vi "Triggers Routing.vi"(7 "Function":enum16{"Connect routes", "Disconnect routes"}(ring), 8 "error in (no error)":errorcluster) -> (0 "error out (no error)":errorcluster)   [LabVIEW 2013]
uses:
  Typedefs/HW config states enum.ctl
  <vilib>/Utility/error.llb/DialogType.ctl
  Global Variables/General Globals.vi
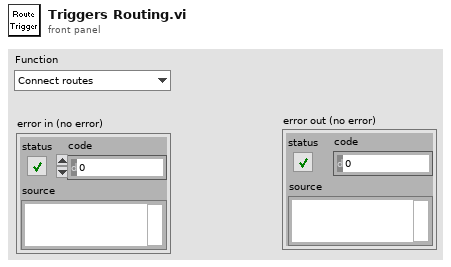
[diagram p1: front panel]
types:
  T1 = typedef "HW config states enum.ctl" = enum16{"Load from file", "Save to file", "Write all", "Read all", "Write XY stage settings", "Write DAQ FPGA settings", "Write Control FPGA settings", "Write Phys Channels", "Clear", "Compare from file"}
  T2 = typedef "Sys Configuration.ctl" = cluster{"XY Stage":T3, "DAQ FPGA":T4, "Control system":T8, "Encoder":T9, "DAQmx Chan":T10, "Computer MAC address":string, "Cam VidRec":T11, "Externalise Triggers":bool, "Laser wavelength (nm)":dbl}
  T3 = typedef "XY Stage config cluster.ctl" = cluster{"COM port":refnum<visa-resource-name>, "XY stage available":bool}
  T4 = typedef "DAQ FPGA config cluster.ctl" = cluster{"Ref":T5, "Target":T6, "Clock Freq (MHz) ":dbl, "input card type":T7, "Samples Wait after Trigger":u16, "AOD fill":u16, "StartupDelay":i32, "Slip Cycle (clock cycles)":u32, "Add Cycle":bool}
  T5 = typedef "FPGA Ref.ctl" = refnum<k20>
  T6 = typedef "nirio_resource_hc.ctl" = tag
  T7 = typedef "FPGA input type AC-DC.ctl" = enum16{"AC Card", "DC Card"}
  T8 = typedef "CTRL system config cluster.ctl" = cluster{"Ethernet opened":bool, "Ethernet Port":u32, "Ctrl FPGA available":bool, "Ctrl FPGA Clock (MHz)":dbl, "Ctrl system MAC address":string, "Control system.Network adapter name":string, "AOD 1 Amplitude":i16, "AOD 2 Amplitude":i16, "AOD 3 Amplitude":i16, "AOD 4 Amplitude":i16, "Data Time Interval (ns)":dbl, "T0 (ns)":dbl, "Ta (ns)":dbl}
  T9 = typedef "Encoder config cluster.ctl" = cluster{"IP address":string, "Port":u16, "Encoder available":bool, "Wheel radius (cm)":dbl}
  T10 = typedef "DAQmx physical channels cluster.ctl" = cluster{"Pockels AO":tag, "Hard shutter AO":tag, "PMT AOs":tag, "Power meter AI":tag}
  T11 = typedef "Cam VidRec HW config setup cluster.ctl" = cluster{"DO flag-Video record":tag, "DO flag-Trial start":tag, "VidRec available":bool}
  T12 = cluster{"PXI backplane trigger":tag, "PXI-6535 terminal to output trigger on":tag}[]
  T13 = typedef "Triggers output setup.ctl" = T14[]
  T14 = typedef "Trigger setup element cluster.ctl" = cluster{"Name":string, "Output?":bool, "Output terminal":tag, "PXI backplane line":tag, "Pulse width (us)":u16}
  T15 = typedef "DialogType.ctl" = u16
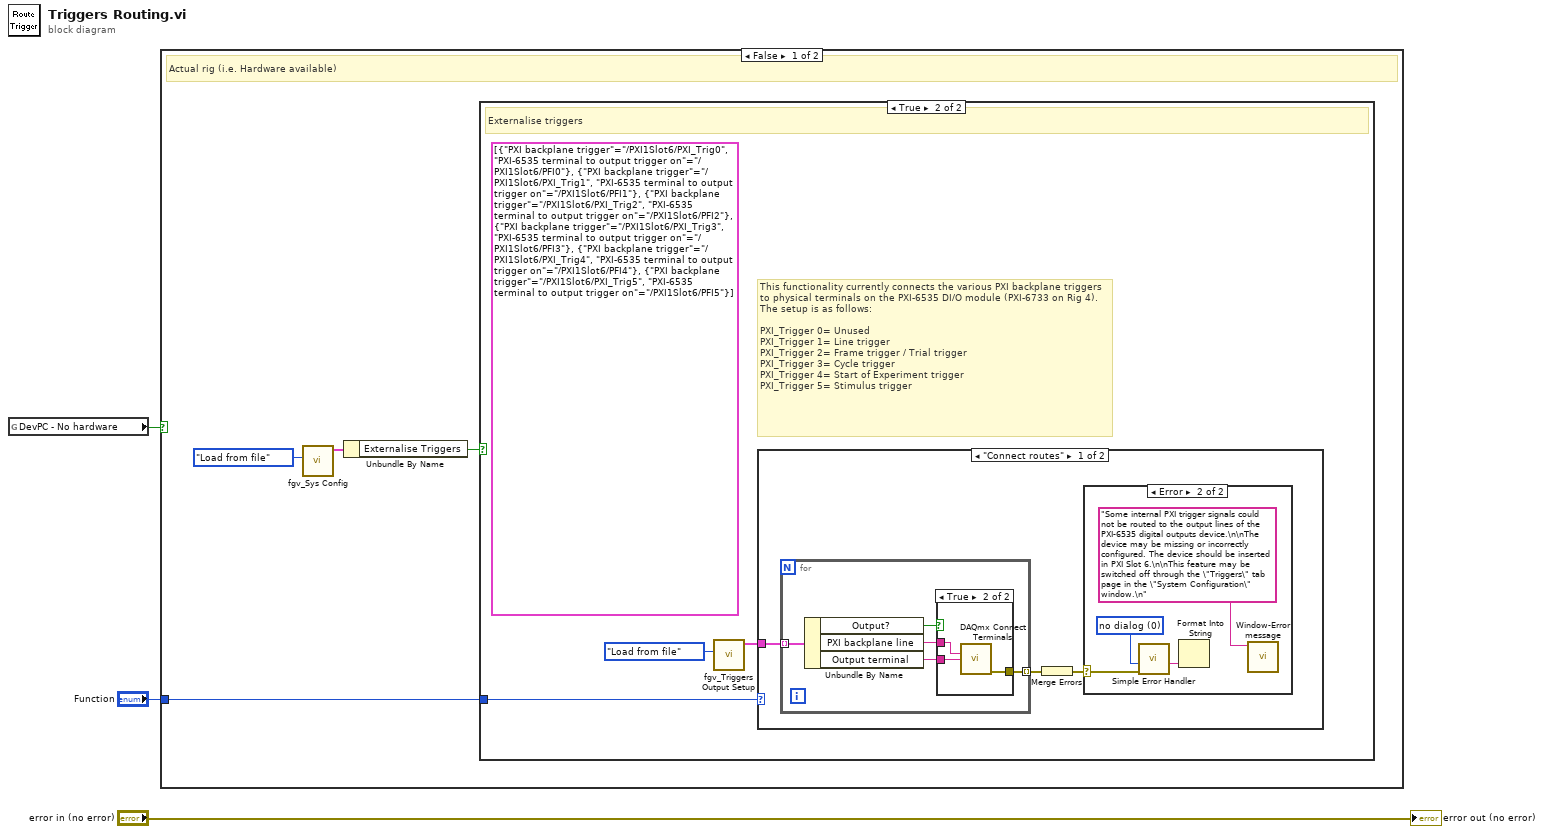
[diagram p0: block diagram]
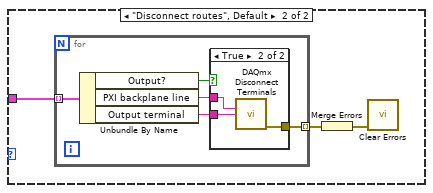
[diagram p5: hidden frame]
diagram:
  n1 = global read "General Globals.vi" "DevPC - No hardware"() -> (w1:bool)
  n2 = case shown="False" w1 {
    tunnel: "Function" -> [w4 _]
    frame False {
      # "Actual rig (i.e. Hardware available)"
      n3 = call "fgv_Sys Config.vi"("Function"=HW_config_states_enum."Load from file") -> ("System Config out"=w6:T2)  [unwired: 9 in, 1 out]
      n4 = Unbundle By Name(w6) -> ("Externalise Triggers"=w5:bool)
      n5 = case shown="True" w5 {
        tunnel: w4 -> [_ w8]
        frame False {
          # "\"Externalise triggers\" is OFF"
        }
        frame True {
          (unwired) T12 [{"PXI backplane trigger"="/PXI1Slot6/PXI_Trig0", "PXI-6535 terminal to output trigger on"="/PXI1Slot6/PFI0"}, {"PXI backplane trigger"="/PXI1Slot6/PXI_Trig1", "PXI-6535 terminal to output trigger on"="/PXI1Slot6/PFI1"}, {"PXI backplane trigger"="/PXI1Slot6/PXI_Trig2", "PXI-6535 terminal to output trigger on"="/PXI1Slot6/PFI2"}, {"PXI backplane trigger"="/PXI1Slot6/PXI_Trig3", "PXI-6535 terminal to output trigger on"="/PXI1Slot6/PFI3"}, {"PXI backplane trigger"="/PXI1Slot6/PXI_Trig4", "PXI-6535 terminal to output trigger on"="/PXI1Slot6/PFI4"}, {"PXI backplane trigger"="/PXI1Slot6/PXI_Trig5", "PXI-6535 terminal to output trigger on"="/PXI1Slot6/PFI5"}] ("Routes mapping array")
          # "This functionality currently connects the various PXI backplane triggers to physical terminals on the PXI-6535 DI/O module (PXI-6733 on Rig 4). The setup is as follows:\n\nPXI_Trigger 0= Unused\nPXI_Trigger 1= Line trigger\nPXI_Trigger 2= Frame trigger / Trial trigger\nPXI_Trigger 3= Cycle trigger\nPXI_Trigger 4= Start of Experiment trigger\nPXI_Trigger 5= Stimulus trigger"
          # "Externalise triggers"
          n6 = call "fgv_Triggers Output Setup.vi"("Function"=HW_config_states_enum."Load from file") -> ("Triggers output setup"=w10:T13)  [unwired: 9 in, 1 out]
          n7 = case shown="\"Connect routes\"" w8 {
            tunnel: w10 -> [w11 w26]
            frame "Connect routes" {
              n8 = for {
                tunnel: [w22] -> w13 mode=indexing
                tunnel: w11 -> [w19] mode=indexing
                n9 = Unbundle By Name(w19) -> ("Output?"=w18:bool, "PXI backplane line"=w21:tag, "Output terminal"=w20:tag)
                n10 = case shown="True" w18 {
                  tunnel: [_ w25] -> w22
                  tunnel: w21 -> [_ w24]
                  tunnel: w20 -> [_ w23]
                  frame False {
                  }
                  frame True {
                    n11 = call <vilib>:"DAQmx Connect Terminals.vi"("source terminal"=w24, "destination terminal"=w23) -> ("error out"=w25:errorcluster)  [unwired: 13 in]
                  }
                }
              }
              n12 = Merge Errors(w13) -> (w12:errorcluster)
              n13 = case shown="Error" w12 {
                selector: w12 -> [_ w15]
                frame No Error {
                }
                frame Error {
                  w17 = T15 0 items=["no dialog", "OK message", "continue or stop message", "OK message + warnings", "continue/stop + warnings"] ("type of dialog (OK msg:1)")
                  n14 = call <vilib>:"Simple Error Handler.vi"("type of dialog (OK msg:1)"=w17, "error in (no error)"=w15) -> ("source out"=w16:string)  [unwired: 3 in, 4 out]
                  n15 = Format Into String(w16) -> ()  [unwired: 3 in, 2 out]
                  n16 = call "Window-Error message.vi"("Message"="Some internal PXI trigger signals could not be routed to the output lines of the PXI-6535 digital outputs device.\n\nThe device may be missing or incorrectly configured. The device should be inserted in PXI Slot 6.\n\nThis feature may be switched off through the \"Triggers\" tab page in the \"System Configuration\" window.\n" ("format string")) -> ()  [unwired: 10 in, 1 out]
                }
              }
            }
            frame "Disconnect routes", Default {
              n17 = for {
                tunnel: [w33] -> w28 mode=indexing
                tunnel: w26 -> [w30] mode=indexing
                n18 = Unbundle By Name(w30) -> ("Output?"=w29:bool, "PXI backplane line"=w32:tag, "Output terminal"=w31:tag)
                n19 = case shown="True" w29 {
                  tunnel: [_ w36] -> w33
                  tunnel: w32 -> [_ w35]
                  tunnel: w31 -> [_ w34]
                  frame False {
                  }
                  frame True {
                    n20 = call <vilib>:"DAQmx Disconnect Terminals.vi"("source terminal"=w35, "destination terminal"=w34) -> ("error out"=w36:errorcluster)  [unwired: 13 in]
                  }
                }
              }
              n21 = Merge Errors(w28) -> (w27:errorcluster)
              n22 = call <vilib>:"Clear Errors.vi"("error in (no error)"=w27) -> ()  [unwired: 6 in, 1 out]
            }
          }
        }
      }
    }
    frame True {
      # "Development Computer (i.e. No hardware available)"
    }
  }
  "error out (no error)" <- "error in (no error)"
